vi "Read_from_server.vi"() -> ()   [LabVIEW 2023]
panel:
  in  "Time interval":u32=1000
  in  "File header if log file is empty":string
  out "Data written to file":string
  in  "Number of tags to read from":i32
  out "Tags choosen to read from":string[](array[string])
  in  "File to save data to":path
  in  "Stop Button":bool
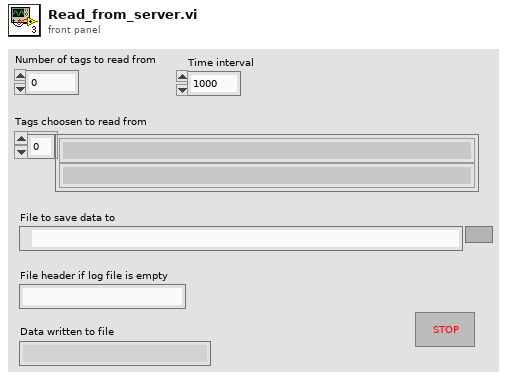
[diagram p1: front panel]
types:
  T1 = enum16{"Read", "Write", "ReadWrite", "BufferedRead", "BufferedReadWrite"}
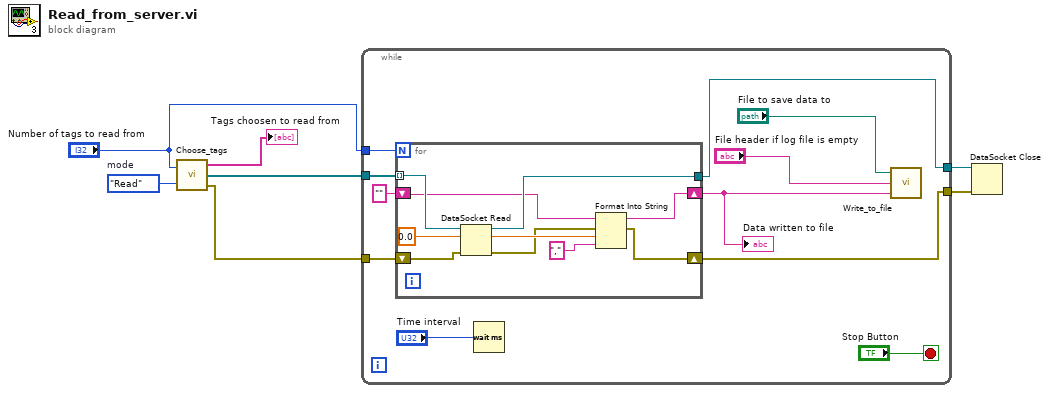
[diagram p0: block diagram]
diagram:
  w4 = T1."Read"  # mode
  n1 = call "Choose_tags.vi"("Number of tags to read from"="Number of tags to read from", "mode"=w4) -> ("Tags opened"=→"Tags choosen to read from":string[], "Opened tags refnumbers"=w2:refnum<k13>[], "error out"=w1:errorcluster)
  n2 = while {
    tunnel: [w12] -> w7
    tunnel: [w15] -> w6
    tunnel: "Number of tags to read from" -> [w14]
    tunnel: w2 -> [w13]
    tunnel: w1 -> [w11]
    stop <- "Stop Button" stop-if-true
    n3 = for {
      N: w14 -> [_]
      tunnel: [w28] -> w15
      tunnel: w13 -> [w26] mode=indexing
      shift-right: [w19] -> w12
      shift-left: w11 -> [w25]
      shift-right: [w24] -> w10
      shift-left: "" -> [w22]
      n4 = DataSocket Read(8:w25, 10:0.0, 11:w26) -> (0:w20:errorcluster, 2:w23:dbl, 3:w28:refnum<k13>)  [unwired: 2 in, 4 out]
      n5 = Format Into String "Format Into String"(initial string=w22, error in=w20, w23, ",") -> (resulting string=w24:string, error out=w19:errorcluster)  [unwired: 1 in]
    }
    "Data written to file" <- w10
    n6 = Wait (ms)(milliseconds to wait="Time interval") -> ()  [unwired: 1 out]
    n7 = call "Write_to_file.vi"("Data to be logged"=w10, "File header if log file is empty"="File header if log file is empty", "file path (use dialog)"="File to save data to") -> ()  [unwired: 1 in]
  }
  n8 = DataSocket Close(8:w7, 11:w6) -> ()  [unwired: 1 in, 2 out]
